vi "analog-delay-test.vi"() -> ()   [LabVIEW 2019]
uses:
  <vilib>/Rock Robotics/WPI/ThirdParty/JAS_Junk/TrajLib/TimeInterpDouble_New.vi
  <vilib>/Rock Robotics/WPI/ThirdParty/JAS_Junk/TrajLib/TimeInterpDouble_AddSample.vi
  <vilib>/Rock Robotics/WPI/ThirdParty/JAS_Junk/TrajLib/TimeInterpDouble_GetSample.vi
  <vilib>/Rock Robotics/WPI/ThirdParty/JAS_Junk/TrajLib/TimeInterpDouble_CleanUp.vi
  <vilib>/Rock Robotics/WPI/ThirdParty/JAS_Junk/TrajLib/MathUtil_Interpolate.vi
  <vilib>/Rock Robotics/WPI/ThirdParty/JAS_Junk/TrajLib/MathUtil_Clamp.vi
  <vilib>/gmath/interp.llb/Search Ordered Table.vi
  <vilib>/Rock Robotics/WPI/ThirdParty/JAS_Junk/TrajLib/Trajectory_Library.lvlib
panel:
  out "Delayed Output":dbl=2000.0 format="%12.4f"
  out "Output":dbl=2000.0 format="%12.4f"
  out "Waveform Chart":cluster{dbl, "Output":dbl}(graph)
  out "IsPresent \nin buffer":bool
  in  "Period (ms)":dbl=2000.0
  in  "Delay (ms)":dbl=500.0
  # "ANALOG DELAY TEST"
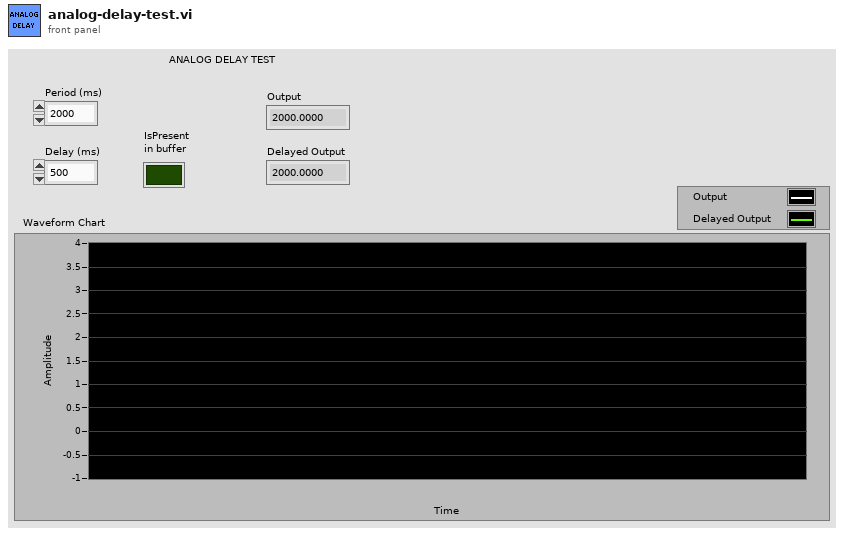
[diagram p1: front panel]
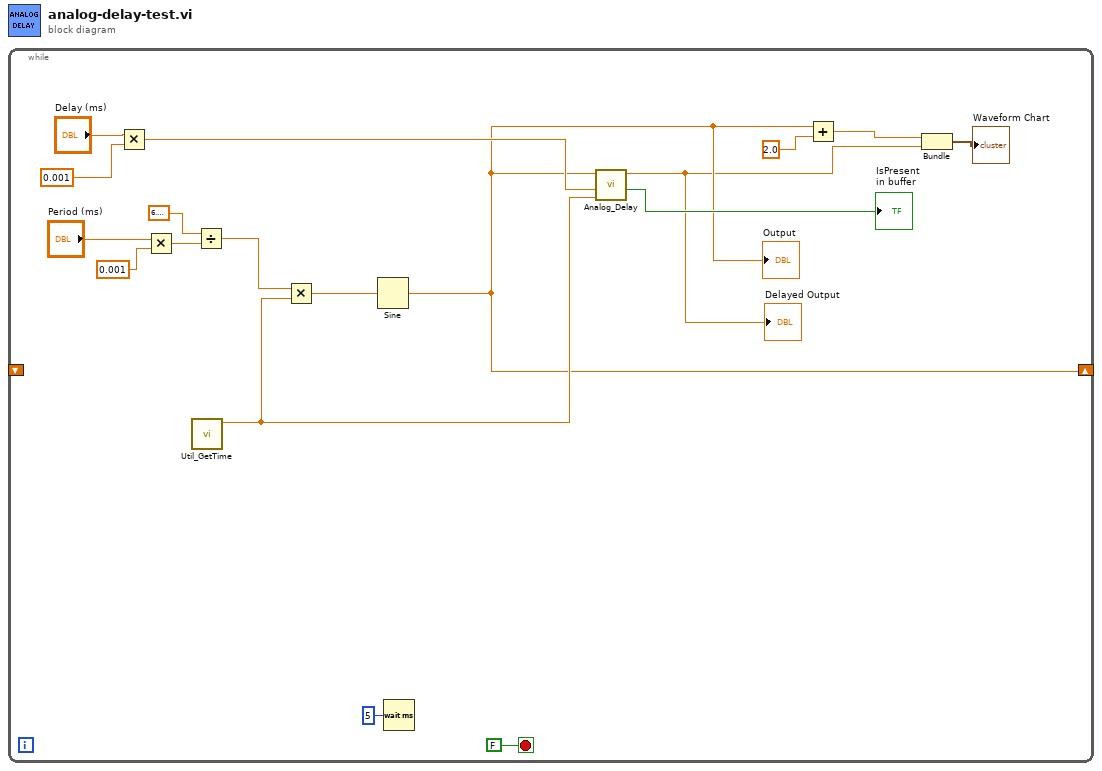
[diagram p0: block diagram]
diagram:
  n1 = while {
    shift-right: [w2] -> _
    shift-left: _ -> [_]
    stop <- FALSE stop-if-true
    n2 = Multiply(x="Delay (ms)", y=0.001) -> (x*y=w13:dbl)
    n3 = Multiply(x="Period (ms)", y=0.001) -> (x*y=w10:dbl)
    n4 = call <vilib>:"Util_GetTime.vi"() -> ("FPGA_Time_Seconds"=w5:dbl)  [unwired: 10 in, 1 out]
    n5 = Divide(x=6.283185307179586, y=w10) -> (x/y=w7:dbl)
    n6 = Multiply(x=w7, y=w5) -> (x*y=w6:dbl)
    n7 = Sine(x=w6) -> (sin(x)=w2:dbl)
    "Output" <- w2
    n8 = Wait (ms)(milliseconds to wait=u32 5) -> ()  [unwired: 1 out]
    n9 = call <vilib>:"Analog_Delay.vi"("Time"=w5, "Delay Time"=w13, "Input"=w2) -> ("IsPresent"=→"IsPresent \nin buffer":bool, "Output"=w1:dbl)  [unwired: 7 in]
    "Delayed Output" <- w1
    n10 = Add(x=w2, y=2.0) -> (x+y=w11:dbl)
    n11 = Bundle(w11, "Output"=w1) -> (→"Waveform Chart":cluster{dbl, "Output":dbl})  [unwired: 1 in]
  }
